vi "Do.vi"(8 "error in":errorcluster, 10 "Actor in":refnum<class "Actor.lvclass">, 11 "Change Blue Laser Rate MSG":refnum<class "Change Blue Laser Rate MSG.lvclass">) -> (0 "error out":errorcluster, 2 "Actor out":refnum<class "Actor.lvclass">)   [LabVIEW 2014, in "eCRDS Library.lvlib" / "Change Blue Laser Rate MSG.lvclass"]
doc: "(<B>Filename</B>: Actor Framework.lvlib:Message.lvclass:Do.vi)\n\nDefines what a message does when it is received by an actor. Generally, a message instructs an actor to invoke one of its methods. By default, this method does nothing. A child class must override it to define behavior. Create a child class by using the Actor Framework Message Maker dialog box."
uses:
  Change Blue Laser Rate MSG.lvclass
  <vilib>/ActorFramework/Actor/Actor.lvclass
  Change Blue Laser Rate MSG.lvclass/Change Blue Laser Rate MSG.ctl
  Instr Actor.lvclass
  CRDS/Commands/Reset Blue Rep Rate/Reset Blue Laser Rep Rate.lvclass
  CRDS/Commands/Reset Blue Rep Rate/Reset Blue Laser Rep Rate.lvclass/Reset Blue Laser Rep Rate.ctl
  SuperActor/Ex Nested.lvclass/Ex Nested.ctl
  Controller/Messages/Update CVT/Update CVT Data.lvclass
  Controller/Messages/Update CVT/Update CVT Data.lvclass/Update CVT Data.ctl
  Controller/Messages/Update CVT/Write Data.vi
  Controller/Messages/Update CVT/Write Group.vi
  Controller/Messages/Update CVT/Write tag.vi
  SuperActor/Read Log Session.vi
  <userlib>/_Session Fwk/Session - Root.lvclass
  reusable/Command/Command.lvclass
  reusable/Session APIs/Session Log/System Log.lvclass
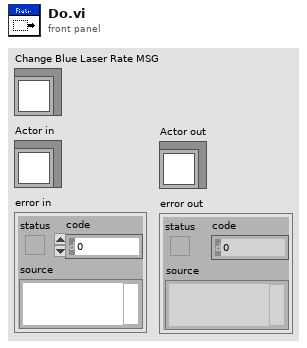
[diagram p1: front panel]
types:
  T1 = typedef "Session - Root.lvclass/Session Handle.ctl" = refnum<data-value>
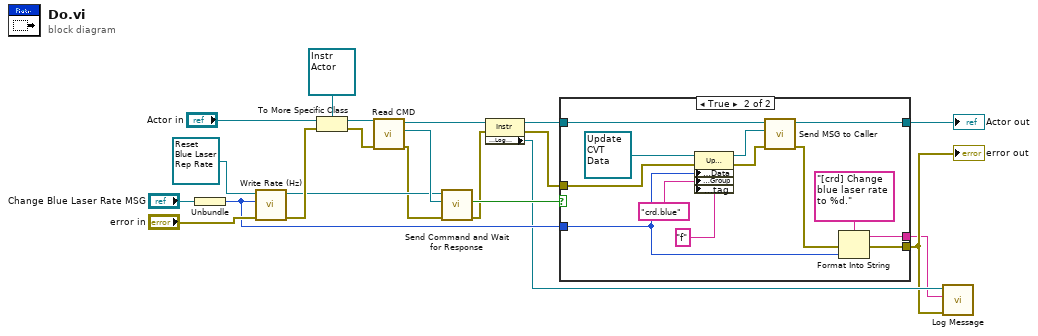
[diagram p0: block diagram]
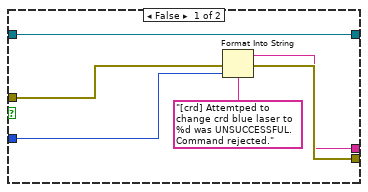
[diagram p2: hidden frame]
diagram:
  n1 = Unbundle("Change Blue Laser Rate MSG") -> (w9:i32)
  n2 = call "Write Rate (Hz).vi"("error in"="error in", "Rate (Hz)"=w9, "Reset Blue Laser Rep Rate in"=refnum<class "Reset Blue Laser Rep Rate.lvclass"> refnum ("Reset Blue Laser Rep Rate.lvclass")) -> ("error out"=w15:errorcluster, "Reset Blue Laser Rep Rate out"=w12:refnum<class "Reset Blue Laser Rep Rate.lvclass">)  [unwired: 7 in]
  n3 = To More Specific Class(target class=refnum<class "Instr Actor.lvclass"> refnum ("Instrument Lib:Instr"), reference="Actor in", error in=w15) -> (specific class reference=w19:refnum<class "Instr Actor.lvclass">, error out=w14:errorcluster)
  n4 = call "Read CMD.vi"("error in (no error)"=w14, "Instr Actor in"=w19) -> ("error out"=w11:errorcluster, "CMD"=w13:refnum<queue>, "Instr Actor out"=w7:refnum<class "Instr Actor.lvclass">)  [unwired: 7 in]
  n5 = call "Send Command and Wait for Response.vi"("error in"=w11, "cmd queue"=w13, "CMD in"=w12) -> ("error out"=w5:errorcluster, "cmd good?"=w10:bool)  [unwired: 6 in, 1 out]
  n6 = property class="Instr"(reference=w7, error in=w5) -> (reference out=w6:refnum<class "Instr Actor.lvclass">, error out=w2:errorcluster, "Accessors:Log Session"=w4:T1)
  n7 = case shown="True" w10 {
    tunnel: w9 -> [w26 w32]
    tunnel: w6 -> [w27 w36]
    tunnel: [w27 w35] -> w8
    tunnel: w2 -> [w24 w34]
    tunnel: [w23 w28] -> w3
    tunnel: [w22 w30] -> w1
    frame False {
      n8 = Format Into String(format string="[crd] Attemtped to change crd blue laser to %d was UNSUCCESSFUL.  Command rejected.", error in=w24, w26) -> (resulting string=w22:string, error out=w23:errorcluster)  [unwired: 1 in]
    }
    frame True {
      n9 = property class="Update CVT Data"(reference=refnum<class "Update CVT Data.lvclass"> refnum ("Controller.lvlib:Update CVT Data"), error in=w34, "Accessors:Data"=w32, "Accessors:Group"="crd.blue" ("Group"), "Accessors:tag"="f" ("tag")) -> (reference out=w37:refnum<class "Update CVT Data.lvclass">, error out=w33:errorcluster)
      n10 = call "Send MSG to Caller.vi"("error in"=w33, "Message"=w37, "Instr in"=w36) -> ("error out"=w29:errorcluster, "Instr out"=w35:refnum<class "Instr Actor.lvclass">)  [unwired: 7 in]
      n11 = Format Into String(format string="[crd] Change blue laser rate to %d.", error in=w29, w32) -> (resulting string=w30:string, error out=w28:errorcluster)  [unwired: 1 in]
    }
  }
  "error out" <- w3
  "Actor out" <- w8
  n12 = call "Log Message.vi"("error in"=w3, "MSG In"=w1, "session in"=w4) -> ()  [unwired: 7 in, 2 out]
